vi "Get Named Range Values (VAR).vi"(8 "error in":errorcluster, 9 "Sheet Name":string, 10 "Named Range Identifier":string, 11 "SpreadsheetDoc in":refnum<k24>) -> (0 "error out":errorcluster, 2 "Cells":variant[][](array[variant]), 3 "SpreadsheetDoc out":refnum<k24>)   [LabVIEW 2019, in "Open Xml.lvlib"]
uses:
  Open Xml.lvlib
  D:/git/Open-Xml-LabVIEW/Source/DocumentFormat.OpenXml.dll
  DocumentFormat.OpenXml.dll
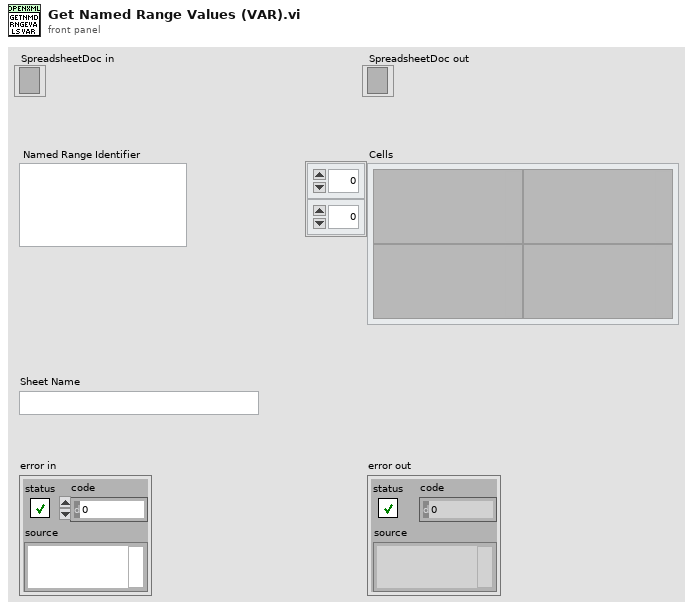
[diagram p1: front panel]
types:
  T1 = typedef "Open Xml.lvlib/Cell DataType.ctl" = enum16{"Void", "Boolean", "Number", "Error", "SharedString", "String", "InlineString", "Date"}
  T2 = cluster{"Number":dbl, "String":string, "Boolean":bool, "Time Stamp":timestamp, "Error":errorcluster}[][]
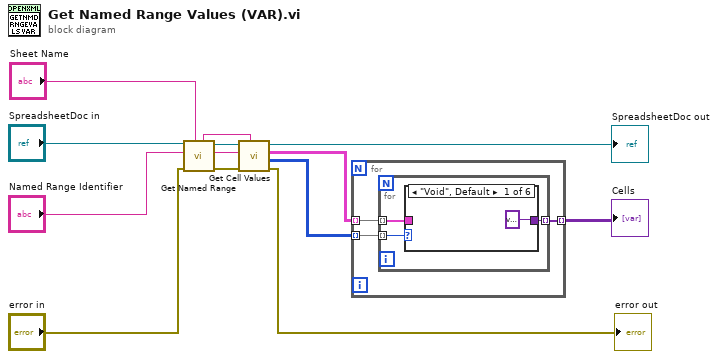
[diagram p0: block diagram]
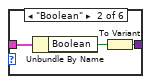
[diagram p2: hidden frame]
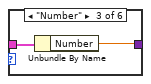
[diagram p3: hidden frame]
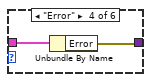
[diagram p4: hidden frame]
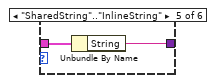
[diagram p5: hidden frame]
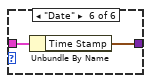
[diagram p6: hidden frame]
diagram:
  n1 = call "Get Named Range.vi"("Sheet Name"="Sheet Name", "error in"="error in", "Range Identifier"="Named Range Identifier", "SpreadsheetDoc in"="SpreadsheetDoc in") -> ("error out"=w9:errorcluster, "Range"=w5:string, "SpreadsheetDoc out"=w7:refnum<k24>, "Sheet Name"=w6:string)  [unwired: 4 in]
  n2 = call "Get Cell Values.vi"("Sheet Name"=w6, "error in"=w9, "Cell Addresses"=w5, "SpreadsheetDoc in"=w7) -> ("error out"=→"error out":errorcluster, "Types"=w2:T1[][], "Cell Values"=w4:T2, "SpreadsheetDoc out"=→"SpreadsheetDoc out":refnum<k24>)  [unwired: 4 in]
  n3 = for {
    tunnel: w4 -> [w16] mode=indexing
    tunnel: w2 -> [w15] mode=indexing
    tunnel: [w14] -> w1 mode=indexing
    n4 = for {
      tunnel: w16 -> [w18] mode=indexing
      tunnel: w15 -> [w19] mode=indexing
      tunnel: [w17] -> w14 mode=indexing
      n5 = case shown="\"Void\", Default" w19 {
        tunnel: w18 -> [_ w23 w25 w27 w29 w31]
        tunnel: [variant ("Variant") w21 w24 w26 w28 w30] -> w17
        frame "Void", Default {
        }
        frame "Boolean" {
          n6 = Unbundle By Name(w23) -> ("Boolean"=w22:bool)
          n7 = To Variant(anything=w22) -> (Variant=w21:variant)
        }
        frame "Number" {
          n8 = Unbundle By Name(w25) -> ("Number"=w24:dbl)
        }
        frame "Error" {
          n9 = Unbundle By Name(w27) -> ("Error"=w26:errorcluster)
        }
        frame "SharedString".."InlineString" {
          n10 = Unbundle By Name(w29) -> ("String"=w28:string)
        }
        frame "Date" {
          n11 = Unbundle By Name(w31) -> ("Time Stamp"=w30:timestamp)
        }
      }
    }
  }
  "Cells" <- w1
